vi "final code Two Tank Liquid Level system .vi"() -> ()   [LabVIEW 2019]
uses:
  <vilib>/addons/control/pid/pid.llb/PID Gain Unit.ctl
  <vilib>/addons/control/pid/pid.llb/PID Time Unit.ctl
  <vilib>/addons/control/pid/pid.llb/PID Structure.ctl
  <vilib>/MakerHub/LINX/Public/Peripherals/PWM/PWM Set Duty Cycle 1 Chan.vi
  <vilib>/MakerHub/LINX/Public/Peripherals/Digital/Digital Write 1 Chan.vi
  <vilib>/MakerHub/LINX/Public/Peripherals/Digital/Digital Write N Chans.vi
  <vilib>/MakerHub/LINX/Private/Local IO/LinxDigitalWrite.vi
  <vilib>/MakerHub/LINX/Public/Utilities/Check Channel.vi
  <vilib>/MakerHub/LINX/Public/Utilities/Open Serial.vi
  <vilib>/addons/control/pid/pid.llb/PID Structure Conversion (DBL).vi
  <vilib>/MakerHub/LINX/Private/Utilties/Generate Error.vi
  <vilib>/addons/control/pid/pid.llb/PID Advanced (DBL).vi
  <vilib>/MakerHub/LINX/Public/Peripherals/PWM/PWM Set Duty Cycle N Chans.vi
  <vilib>/MakerHub/LINX/LMH-LINX.lvlib
  <vilib>/MakerHub/LINX/Public/Sensors/Distance/Ultrasonic/Ultrasonic.lvlib
  <vilib>/addons/control/pid/NI_PID_pid.lvlib
  <vilib>/httpClient/LabVIEWHTTPClient.lvlib
panel:
  out "Phase portrait":cluster{"X":dbl, "Y":dbl}[](graph)
  out "Centimeters":dbl
  out "Water Level":dbl(slide) scale=0.0..16.0
  out "led brightness":dbl(slide) scale=0.0..0.5
  in  "pump default speed":dbl
  out "Waveform Chart":cluster{"Setpoint":dbl, "Centimeters":dbl}(graph)
  out "Setpoint":dbl(slide) scale=0.0..16.0
  in  "Setpoint":dbl
  in  "Manual overide pompe":dbl(slide) scale=0.0..100.0
  in  "Manual":bool
  in  "output range":cluster{"output high":dbl, "output low":dbl}={"output high"=100.0, "output low"=0.0} {"output low" min=0.0 max=2500.0 format="%.2f"; "output high" min=0.0 max=2500.0 format="%.2f"}
  out "PID output":dbl format="%.1f"
  in  "setpoint range":cluster{"setpoint high":dbl, "setpoint low":dbl}={"setpoint high"=60.0, "setpoint low"=0.0} {"setpoint high" min=0.0 max=60.0 format="%.2f"; "setpoint low" min=0.0 max=60.0 format="%.2f"}
  in  "Initialize":bool
  out "PID (dt) 2":dbl
  in  "PID (dt)":dbl
  in  "Proportional":dbl=5.0 format="%#.10f"
  in  "Integral":dbl=0.008 format="%#.3g"
  in  "Derivative":dbl format="%#.3g"
  in  "PID Topology":T1 items=["Academic (Standard)", "Parallel", "Series"]
  in  "Integral Unit":T2 items=["min", "s"]
  in  "Derivative Unit":T2 items=["min", "s"]
  in  "Proportional Unit":T3 items=["Gain (Kc)", "Band (PB)"]
  out "Device Name":string
  in  "direction1":bool
  in  "direction2":bool
  in  "stop":bool
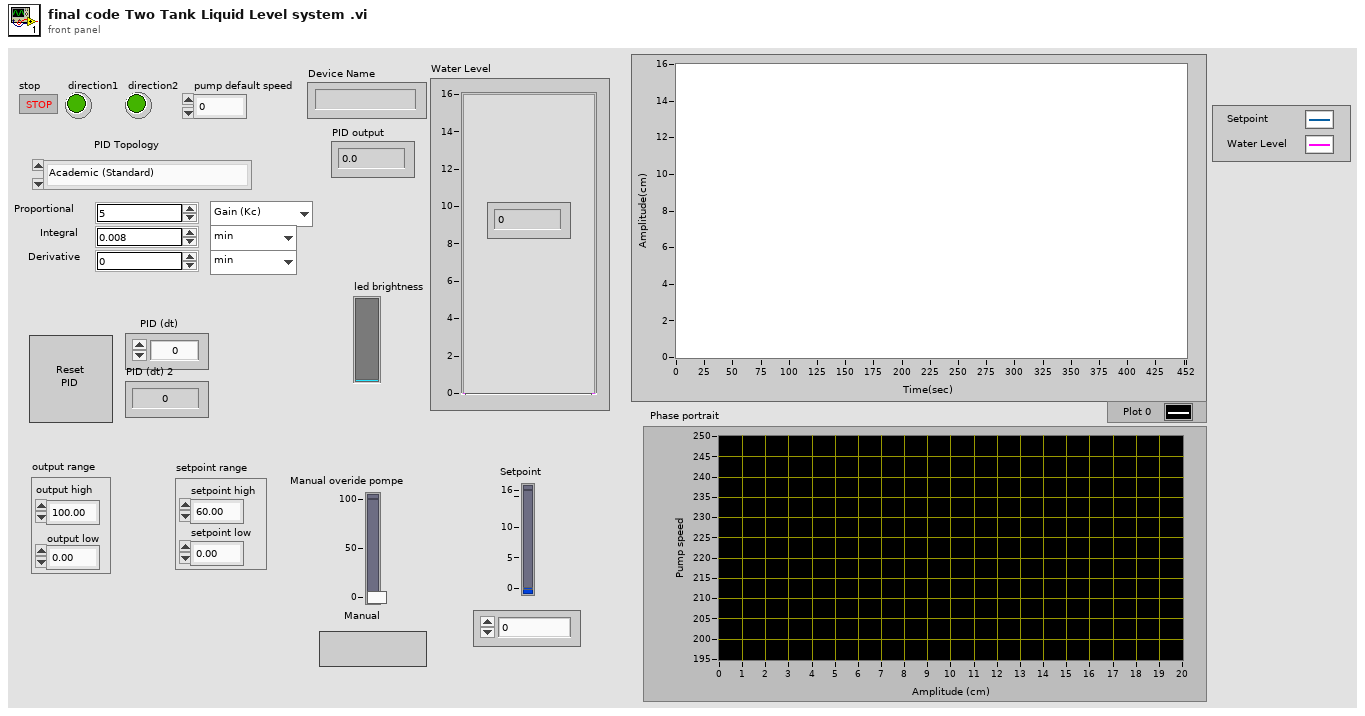
[diagram p1: front panel]
types:
  T1 = typedef "NI_PID_pid.lvlib/PID Structure.ctl" = u16
  T2 = typedef "NI_PID_pid.lvlib/PID Time Unit.ctl" = u16
  T3 = typedef "NI_PID_pid.lvlib/PID Gain Unit.ctl" = u16
  T4 = typedef "LMH-LINX.lvlib/LINX Ref.ctl" = cluster{"IO":T5, "Interface":T6, "LINX Device Config":T7}
  T5 = typedef "LMH-LINX.lvlib/Platform.ctl" = enum16{"Remote", "Local"}
  T6 = typedef "LMH-LINX.lvlib/Interface.ctl" = enum16{"Serial", "TCP"}
  T7 = typedef "LMH-LINX.lvlib/Device.lvlib/LINX Device Config.ctl" = cluster{"Interface":T6, "COM Port":refnum<visa-resource-name>, "TCP Configuration":T8, "Device Family":u8, "Device ID":u8, "Device Name":string, "TCP Ref":refnum<k5>, "Channels":T9}
  T8 = typedef "LMH-LINX.lvlib/Device.lvlib/TCP Config.ctl" = cluster{"IP Address":string, "Port":u16}
  T9 = typedef "LMH-LINX.lvlib/Channels.ctl" = cluster{"DI":u8[], "DO":u8[], "AI":u8[], "AO":u8[], "PWM":u8[], "QE":u8[], "UART":u8[], "I2C 2":u8[], "SPI":u8[], "CAN":u8[], "Servo":u8[], "AI Ref (V)":dbl, "AI Resolution (Bits)":u8, "AO Ref (V)":dbl, "AO Resolution (Bits)":u8}
  T10 = cluster{"proportional gain (Kc)":dbl, "integral time (Ti, min)":dbl, "derivative time (Td, min)":dbl}
  T11 = typedef "LabVIEWHTTPClient.lvlib/ClientHandle.ctl" = refnum<k1>
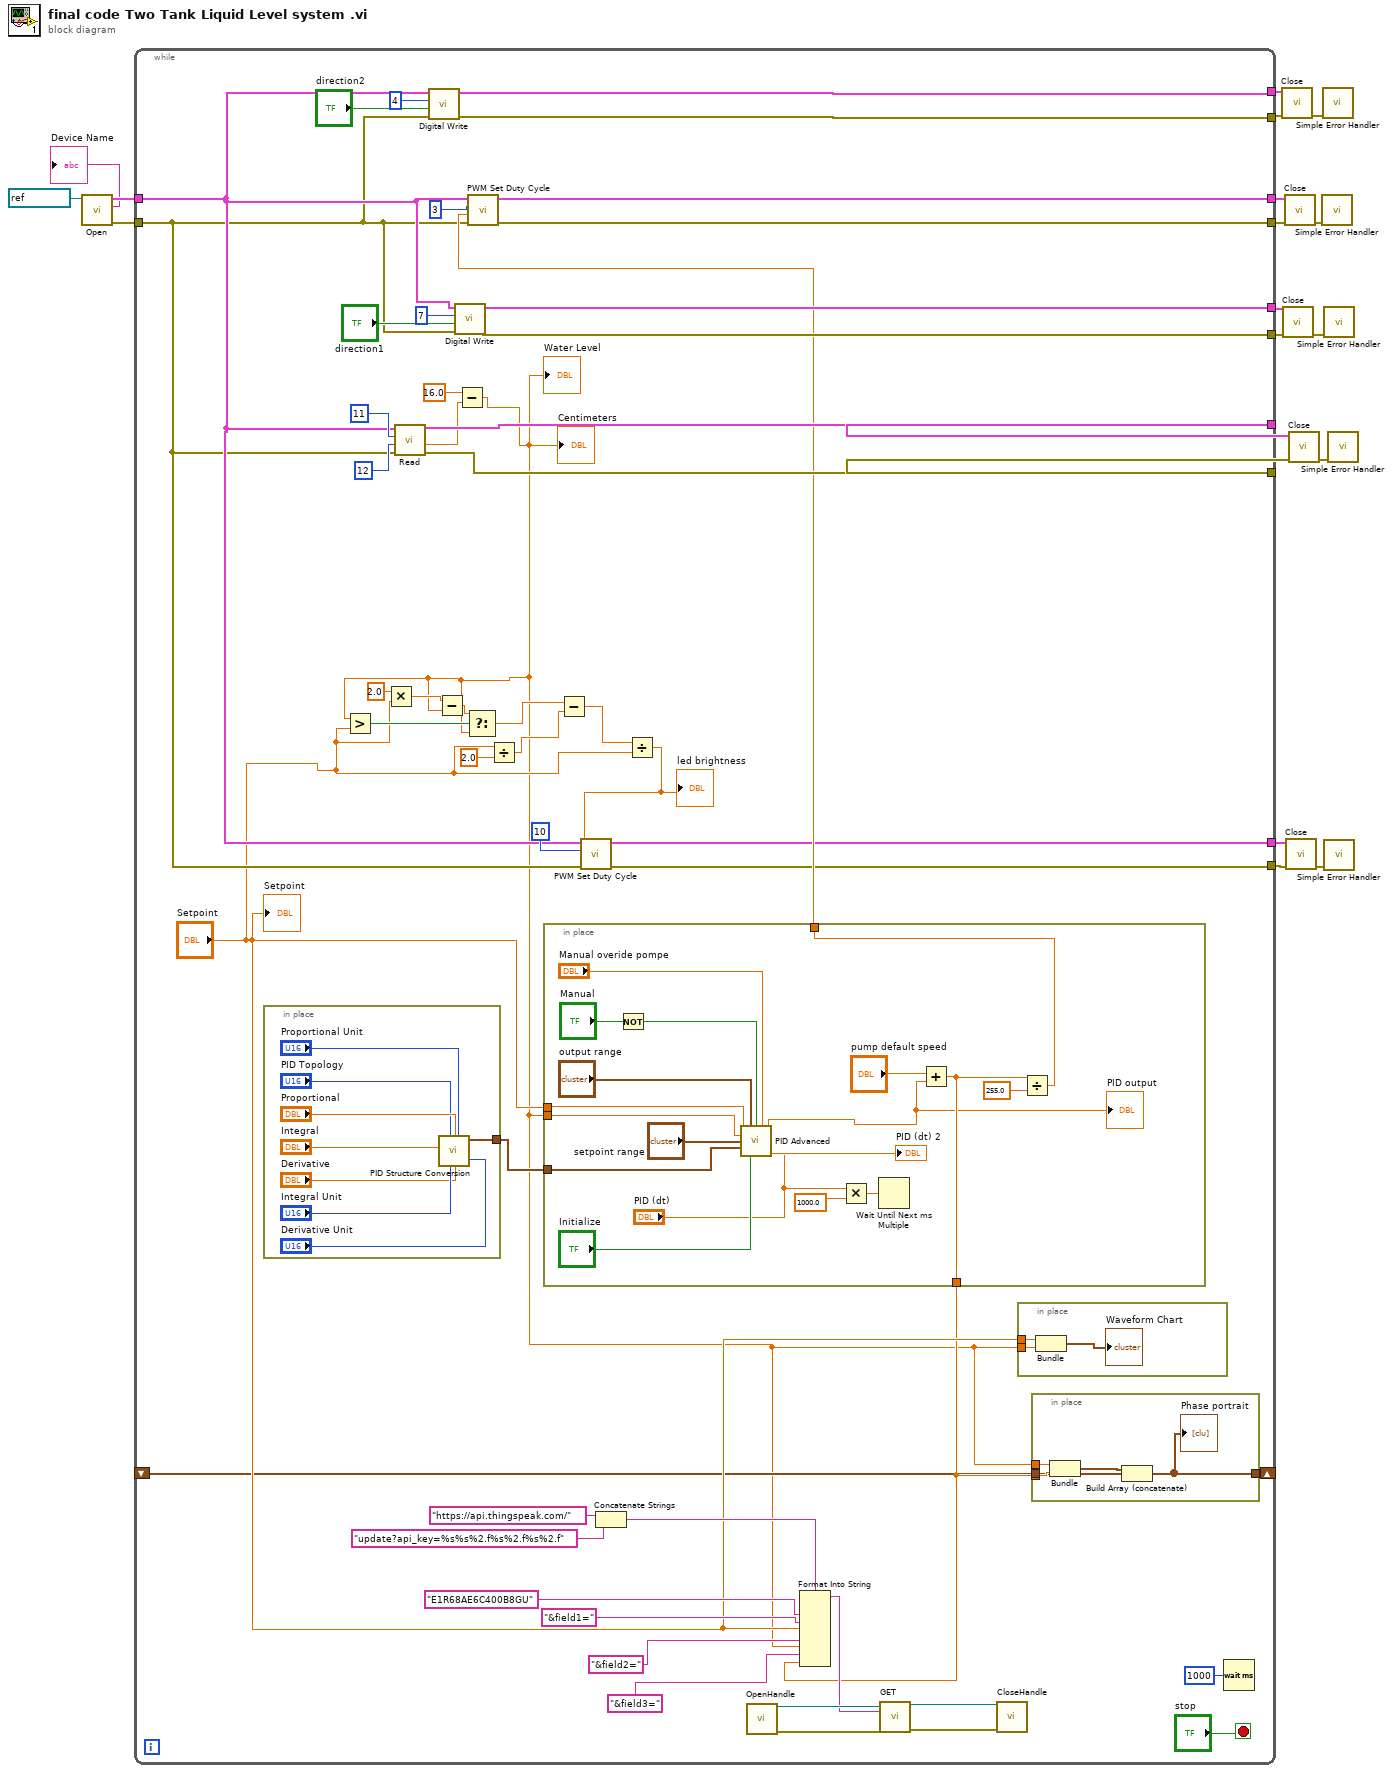
[diagram p0: block diagram]
diagram:
  n1 = call-poly <vilib>:"Open.vi"("Serial Port"=refnum<visa-resource-name> "COM3") -> ("Error Out"=w17:errorcluster, "Device Name"=→"Device Name":string, "LINX Resource"=w18:T4)  [unwired: 8 in]
  n2 = while {
    tunnel: w18 -> [w30]
    tunnel: w17 -> [w29]
    tunnel: [w69] -> w16
    tunnel: [w68] -> w15
    tunnel: [w62] -> w14
    tunnel: [w61] -> w13
    tunnel: [w60] -> w12
    tunnel: [w59] -> w11
    tunnel: [w56] -> w10
    tunnel: [w55] -> w9
    tunnel: [w28] -> w8
    tunnel: [w27] -> w7
    shift-right: [w24] -> _
    shift-left: _ -> [w23]
    stop <- "stop" stop-if-true
    n3 = in-place {
      in-place-border: [w98] -> w54
      n4 = call-poly <vilib>:"PID Structure Conversion.vi"("derivative unit"="Derivative Unit", "proportional unit"="Proportional Unit", "integral unit"="Integral Unit", "PID structure"="PID Topology", "derivative"="Derivative", "integral"="Integral", "proportional"="Proportional") -> ("PID gains"=w98:T10)  [unwired: 4 in]
    }
    n5 = Multiply(x=2.0 ("y"), y="Setpoint") -> (x*y=w37:dbl)
    n6 = call <vilib>:"Read.vi"("Error In"=w29, "DO Channel"=u8 12, "DI Channel"=u8 11, "LINX Resource"=w30) -> ("Error Out"=w55:errorcluster, "Centimeters"=w21:dbl, "LINX Resource"=w56:T4)  [unwired: 4 in, 1 out]
    n7 = call-poly <vilib>:"Digital Write.vi"("Error In"=w29, "Output Value"="direction2", "DO Channel"=u8 4, "LINX Resource"=w30) -> ("Error Out"=w61:errorcluster, "LINX Resource"=w62:T4)  [unwired: 6 in]
    n8 = call-poly <vilib>:"Digital Write.vi"("Error In"=w29, "Output Value"="direction1", "DO Channel"=u8 7, "LINX Resource"=w30) -> ("Error Out"=w59:errorcluster, "LINX Resource"=w60:T4)  [unwired: 6 in]
    n9 = Subtract(x=16.0, y=w21) -> (x-y=w20:dbl)
    "Centimeters" <- w20
    "Water Level" <- w20
    n10 = Greater?(x=w20, y="Setpoint") -> (0:w39:bool)
    n11 = Subtract(x=w37, y=w20) -> (x-y=w36:dbl)
    n12 = Select(t=w36, s=w39, f=w20) -> (s? t:f=w35:dbl)
    n13 = Divide(x="Setpoint", y=2.0) -> (x/y=w33:dbl)
    n14 = in-place {
      in-place-border: w54 -> [w91]
      in-place-border: "Setpoint" -> [w87]
      in-place-border: w20 -> [w88]
      in-place-border: [w81] -> w25
      in-place-border: [w82] -> w53
      n15 = Not(x="Manual") -> (.not. x?=w93:bool)
      n16 = call-poly <vilib>:"PID Advanced.vi"("setpoint"=w87, "output range"="output range", "auto? (T)"=w93, "manual control"="Manual overide pompe", "process variable"=w88, "setpoint range"="setpoint range", "PID gains"=w91, "dt (s)"="PID (dt)", "reinitialize? (F)"="Initialize") -> ("output"=w80:dbl, "dt out (s)"=→"PID (dt) 2":dbl)  [unwired: 5 in]
      "PID output" <- w80
      n17 = Multiply(x="PID (dt)", y=1000.0) -> (x*y=w89:dbl)
      n18 = Wait Until Next ms Multiple(millisecond multiple=w89) -> ()  [unwired: 1 out]
      n19 = Add(x="pump default speed", y=w80) -> (x+y=w81:dbl)
      n20 = Divide(x=w81, y=255.0) -> (x/y=w82:dbl)
    }
    n21 = call-poly <vilib>:"PWM Set Duty Cycle.vi"("Error In"=w29, "Duty Cycle (0-1)"=w53, "PWM Channel"=u8 3 ("DO Channel"), "LINX Resource"=w30) -> ("Error Out"=w69:errorcluster, "LINX Resource"=w68:T4)  [unwired: 6 in]
    n22 = Subtract(x=w35, y=w33) -> (x-y=w32:dbl)
    n23 = Concatenate Strings("https://api.thingspeak.com/" ("string"), "update?api_key=%s%s%2.f%s%2.f%s%2.f" ("string")) -> (w45:string)
    n24 = Divide(x=w32, y="Setpoint") -> (x/y=w31:dbl)
    "led brightness" <- w31
    n25 = call-poly <vilib>:"PWM Set Duty Cycle.vi"("Error In"=w29, "Duty Cycle (0-1)"=w31, "PWM Channel"=u8 10 ("DO Channel"), "LINX Resource"=w30) -> ("Error Out"=w27:errorcluster, "LINX Resource"=w28:T4)  [unwired: 6 in]
    n26 = call <vilib>:"OpenHandle.vi"() -> ("client handle out"=w52:T11, "error out"=w50:errorcluster)  [unwired: 14 in]
    n27 = Format Into String "Format Into String"(format string=w45, "E1R68AE6C400B8GU" ("initial string"), "&field1=", "Setpoint", "&field2=", w20, "&field3=", w25) -> (resulting string=w48:string)  [unwired: 2 in, 1 out]
    n28 = call <vilib>:"GET.vi"("client handle"=w52, "url"=w48, "error in (no error)"=w50) -> ("client handle out"=w51:T11, "error out"=w49:errorcluster)  [unwired: 9 in, 2 out]
    n29 = call <vilib>:"CloseHandle.vi"("client handle"=w51, "error in (no error)"=w49) -> ()  [unwired: 13 in, 1 out]
    n30 = in-place {
      in-place-border: "Setpoint" -> [w77]
      in-place-border: w20 -> [w78]
      n31 = Bundle("Setpoint"=w77, w78) -> (→"Waveform Chart":cluster{"Setpoint":dbl, dbl})  [unwired: 1 in]
    }
    n32 = in-place {
      in-place-border: w20 -> [w75]
      in-place-border: w25 -> [w76]
      in-place-border: [w73] -> w24
      in-place-border: w23 -> [w72]
      n33 = Bundle(w75, w76) -> (w74:cluster{dbl, dbl})  [unwired: 1 in]
      n34 = Build Array (concatenate)(w74, w72) -> (w73:cluster{dbl, dbl}[])
      "Phase portrait" <- w73
    }
    n35 = Wait (ms)(milliseconds to wait=u32 1000) -> ()  [unwired: 1 out]
    "Setpoint" <- "Setpoint"
  }
  n36 = call <vilib>:"Close.vi"("Error In"=w13, "LINX Resource"=w14) -> ("Error Out"=w6:errorcluster)  [unwired: 9 in]
  n37 = call <vilib>:"Close.vi"("Error In"=w11, "LINX Resource"=w12) -> ("Error Out"=w4:errorcluster)  [unwired: 9 in]
  n38 = call <vilib>:"Close.vi"("Error In"=w16, "LINX Resource"=w15) -> ("Error Out"=w5:errorcluster)  [unwired: 9 in]
  n39 = call <vilib>:"Close.vi"("Error In"=w7, "LINX Resource"=w8) -> ("Error Out"=w2:errorcluster)  [unwired: 9 in]
  n40 = call <vilib>:"Close.vi"("Error In"=w9, "LINX Resource"=w10) -> ("Error Out"=w3:errorcluster)  [unwired: 9 in]
  n41 = call <vilib>:"Simple Error Handler.vi"("error in (no error)"=w5) -> ()  [unwired: 4 in, 5 out]
  n42 = call <vilib>:"Simple Error Handler.vi"("error in (no error)"=w6) -> ()  [unwired: 4 in, 5 out]
  n43 = call <vilib>:"Simple Error Handler.vi"("error in (no error)"=w4) -> ()  [unwired: 4 in, 5 out]
  n44 = call <vilib>:"Simple Error Handler.vi"("error in (no error)"=w2) -> ()  [unwired: 4 in, 5 out]
  n45 = call <vilib>:"Simple Error Handler.vi"("error in (no error)"=w3) -> ()  [unwired: 4 in, 5 out]
